vi "Copy_File.vi"(8 "error in (no error)":errorcluster, 9 "newName":string, 10 "sourcePath":path, 11 "AB_Destination in":refnum<class "AB_Destination.lvclass">) -> (0 "error out":errorcluster, 2 "destinationPath":path, 3 "AB_Destination out":refnum<class "AB_Destination.lvclass">)   [LabVIEW 2020, in "AB_Destination.lvclass"]
uses:
  <vilib>/AppBuilder/AB_Classes/Destination/AB_Destination.lvclass
  <vilib>/AppBuilder/AB_Classes/Destination/AB_Destination.lvclass/AB_Destination.ctl
  <resource>/Framework/Providers/Common/provcom_StringGlobals.vi
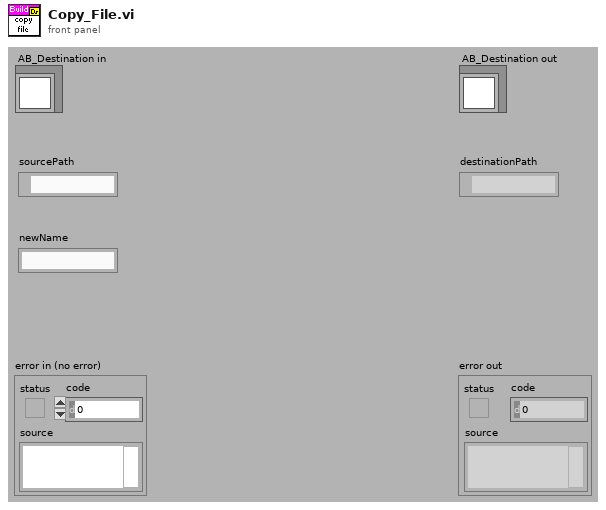
[diagram p1: front panel]
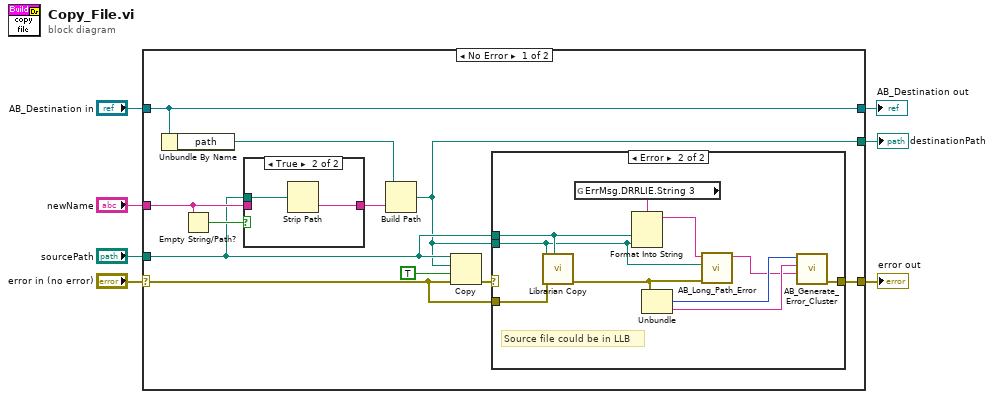
[diagram p0: block diagram]
diagram:
  n1 = case shown="No Error" "error in (no error)" {
    selector: "error in (no error)" -> [w11 w34]
    tunnel: [w12 w34] -> w6
    tunnel: [w18 w33] -> w4
    tunnel: "AB_Destination in" -> [w18 w33]
    tunnel: "sourcePath" -> [w10 _]
    tunnel: "newName" -> [w16 _]
    tunnel: [w9 _] -> w1
    frame No Error {
      n2 = Unbundle By Name(w18) -> ("path"=w14:path)
      n3 = Empty String/Path?(string/path=w16) -> (empty?=w17:bool)
      n4 = case shown="True" w17 {
        tunnel: [w30 w32] -> w15
        tunnel: w16 -> [w30 _]
        tunnel: w10 -> [_ w31]
        frame False {
        }
        frame True {
          n5 = Strip Path(path=w31) -> (name=w32:string)  [unwired: 1 out]
        }
      }
      n6 = Build Path(base path=w14, name or relative path=w15) -> (appended path=w9:path)
      n7 = Copy(8:w11, 9:TRUE ("overwrite (F)"), 10:w9, 11:w10) -> (0:w13:errorcluster)  [unwired: 3 out]
      n8 = case shown="Error" w13 {
        selector: w13 -> [w19 _]
        tunnel: w10 -> [_ w25]
        tunnel: w9 -> [_ w23]
        tunnel: [w19 w28] -> w12
        tunnel: w11 -> [_ w29]
        frame No Error {
        }
        frame Error {
          # "Source file could be in LLB"
          n9 = call <vilib>:"Librarian Copy.vi"("source"=w25, "error in (no error)"=w29, "destination"=w23) -> ("error out"=w22:errorcluster)  [unwired: 2 in, 6 out]
          n10 = global read "provcom_StringGlobals.vi" "ErrMsg.DRRLIE.String 3"() -> (w24:string)
          n11 = Format Into String(format string=w24, w25, w23) -> (resulting string=w21:string)  [unwired: 2 in, 1 out]
          n12 = Unbundle(w22) -> ("code"=w27:i32, "source"=w26:string)  [unwired: 1 out]
          n13 = call <vilib>:"AB_Long_Path_Error.vi"("error in (no error)"=w22, "Path"=w23, "error string in"=w21) -> ("error string out"=w20:string)  [unwired: 7 in, 1 out]
          n14 = call <vilib>:"AB_Generate_Error_Cluster.vi"("Additional Message"=w20, "source"=w26, "Code"=w27) -> ("error out"=w28:errorcluster)  [unwired: 1 in, 7 out]
        }
      }
    }
    frame Error {
    }
  }
  "error out" <- w6
  "AB_Destination out" <- w4
  "destinationPath" <- w1
